vi "MeasurementLink Common Proto Generator.vi"(0 "Proto File Path":path[](array[path]), 1 "Generated Library Name":string, 2 "Library Suffix":string caption="Generated Library Suffix", 3 "Generate":enum16{"gRPC Server", "gRPC Client", "Both"}(ring), 5 "Import Paths":path[](array[path]), 7 "Prototype Library":path, 9 "Target Project":path, 11 "error in (no error)":errorcluster) -> (15 "error out":errorcluster)   [LabVIEW 2020]
uses:
  Generator/_Editor/MeasurementService Editor.lvlib
panel:
  in  "Debug - Prompt before deleting disk content? (F)":bool
  in  "Debug - Leave Project Open? (F)":bool
  # "Ignored for servers as of v0.5.2.2"
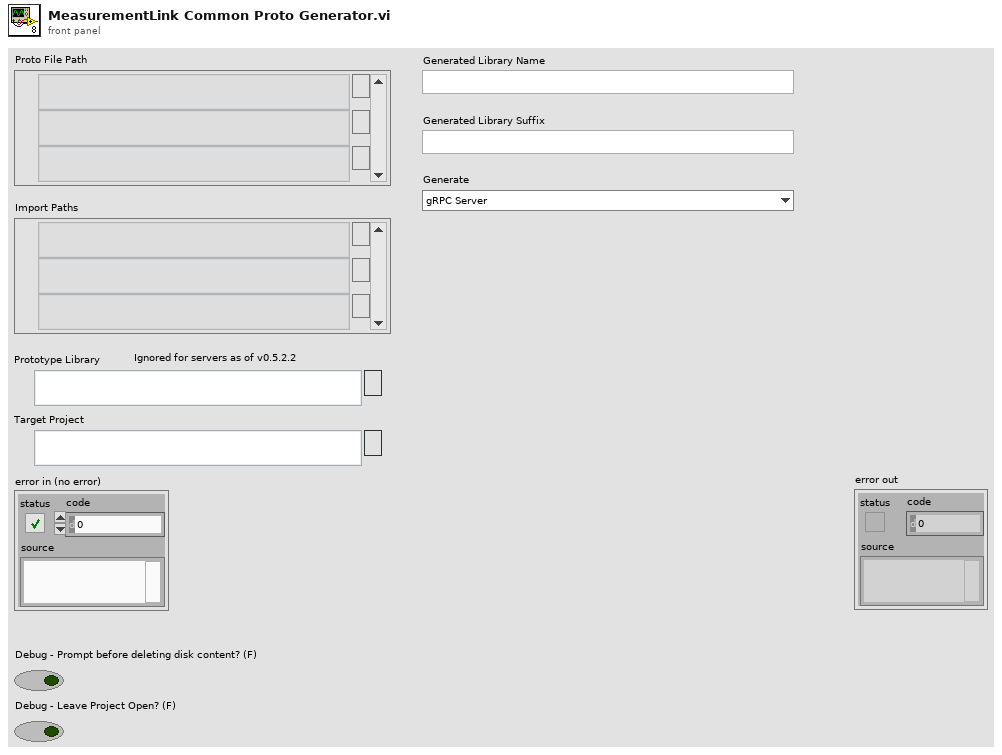
[diagram p1: front panel]
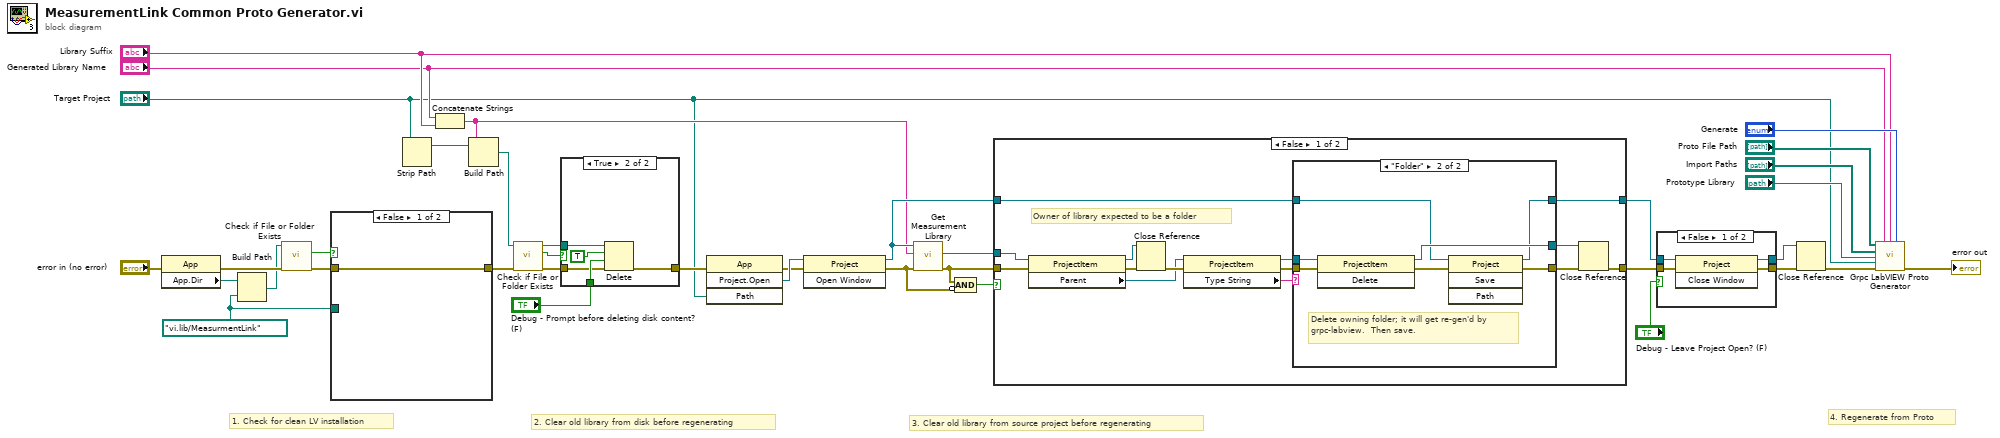
[diagram p0: block diagram]
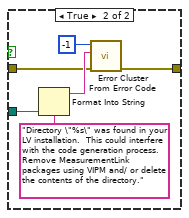
[diagram p2: hidden frame]
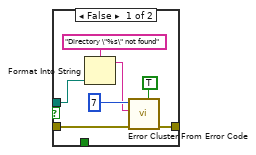
[diagram p3: hidden frame]
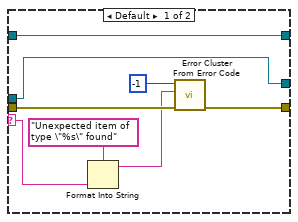
[diagram p4: hidden frame]
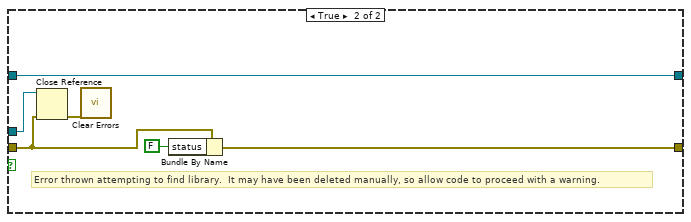
[diagram p5: hidden frame]
diagram:
  w1 = path "vi.lib/MeasurmentLink" ("Target Project")
  # "4. Regenerate from Proto"
  # "3. Clear old library from source project before regenerating"
  # "2. Clear old library from disk before regenerating"
  # "1. Check for clean LV installation"
  n1 = property class="App"(error in="error in (no error)") -> (error out=w6:errorcluster, "App.Dir"=w8:path)  [unwired: 1 in, 1 out]
  n2 = Build Path(base path=w8, name or relative path=w1) -> (appended path=w5:path)
  n3 = call <vilib>:"Check if File or Folder Exists.vi"("error in (no error)"=w6, "path"=w5) -> ("error out"=w3:errorcluster, "file or folder exists?"=w4:bool)  [unwired: 7 in, 1 out]
  n4 = case shown="False" w4 {
    tunnel: w3 -> [w38 w41]
    tunnel: [w38 w42] -> w2
    tunnel: w1 -> [_ w39]
    frame False {
    }
    frame True {
      n5 = Format Into String(format string="Directory \"%s\" was found in your LV installation.  This could interfere with the code generation process.  Remove MeasurementLink packages using VIPM and/ or delete the contents of the directory.", w39) -> (resulting string=w43:string)  [unwired: 2 in, 1 out]
      n6 = call <vilib>:"Error Cluster From Error Code.vi"("error in (no error)"=w41, "error message (\"\")"=w43, "error code (0)"=-1) -> ("error out"=w42:errorcluster)  [unwired: 6 in]
    }
  }
  n7 = Strip Path(path="Target Project") -> (stripped path=w10:path)  [unwired: 1 out]
  n8 = Concatenate Strings("Generated Library Name", "Library Suffix") -> (w26:string)
  n9 = Build Path(base path=w10, name or relative path=w26) -> (appended path=w22:path)
  n10 = call <vilib>:"Check if File or Folder Exists.vi"("error in (no error)"=w2, "path"=w22) -> ("error out"=w21:errorcluster, "file or folder exists?"=w19:bool, "dup path"=w20:path)  [unwired: 7 in]
  n11 = case shown="True" w19 {
    tunnel: [w50 w55] -> w25
    tunnel: "Debug - Prompt before deleting disk content? (F)" -> [_ w54]
    tunnel: w21 -> [w49 w53]
    tunnel: w20 -> [w47 w52]
    frame False {
      n12 = Format Into String(format string="Directory \"%s\" not found", w47) -> (resulting string=w46:string)  [unwired: 2 in, 1 out]
      n13 = call <vilib>:"Error Cluster From Error Code.vi"("is warning? (False)"=TRUE, "error in (no error)"=w49, "error message (\"\")"=w46, "error code (0)"=7) -> ("error out"=w50:errorcluster)  [unwired: 5 in]
    }
    frame True {
      n14 = Delete(path (use dialog)=w52, entire hierarchy (F)=TRUE, confirm (F)=w54, error in=w53) -> (error out=w55:errorcluster)  [unwired: 1 in, 2 out]
    }
  }
  n15 = invoke class="App" method="Project.Open"(error in=w25, "Path"="Target Project") -> (error out=w36:errorcluster, "Project:Open"=w37:refnum<vi>)  [unwired: 2 in, 2 out]
  n16 = invoke class="Project" method="Open Window"(reference=w37, error in=w36) -> (reference out=w27:refnum<vi>, error out=w29:errorcluster)  [unwired: 1 in, 1 out]
  n17 = call "Get Measurement Library.vi"("error in (no error)"=w29, "Measurement Service Name"=w26, "Project in"=w27) -> ("error out"=w23:errorcluster, "Measurement Library Item"=w28:refnum<vi>)  [unwired: 7 in]
  n18 = Compound Arithmetic op=AND(w23, invert w29) -> (w30:bool)
  n19 = case shown="False" w30 {
    tunnel: w28 -> [w69 w88]
    tunnel: w27 -> [w62 w89]
    tunnel: [w59 w89] -> w35
    tunnel: [w58 w91] -> w34
    tunnel: w23 -> [w57 w87]
    frame False {
      # "Owner of library expected to be a folder"
      n20 = property class="ProjectItem"(reference=w69, error in=w57) -> (reference out=w68:refnum<vi>, error out=w70:errorcluster, "Parent"=w66:refnum<vi>)
      n21 = Close Reference(reference=w68, error in (no error)=w70) -> (error out=w67:errorcluster)
      n22 = property class="ProjectItem"(reference=w66, error in=w67) -> (reference out=w63:refnum<vi>, error out=w64:errorcluster, "Type String"=w65:string)
      n23 = case shown="\"Folder\"" w65 {
        selector: w65 -> [w75 _]
        tunnel: w64 -> [w78 w85]
        tunnel: w63 -> [w72 w84]
        tunnel: [w77 w81] -> w61
        tunnel: w62 -> [w71 w80]
        tunnel: [w71 w79] -> w59
        tunnel: [w72 w83] -> w60
        frame Default {
          n24 = Format Into String(format string="Unexpected item of type \"%s\" found", w75) -> (resulting string=w74:string)  [unwired: 2 in, 1 out]
          n25 = call <vilib>:"Error Cluster From Error Code.vi"("error in (no error)"=w78, "error message (\"\")"=w74, "error code (0)"=-1) -> ("error out"=w77:errorcluster)  [unwired: 6 in]
        }
        frame "Folder" {
          # "Delete owning folder; it will get re-gen'd by grpc-labview.  Then save."
          n26 = invoke class="ProjectItem" method="Delete"(reference=w84, error in=w85) -> (reference out=w83:refnum<vi>, error out=w82:errorcluster)  [unwired: 1 in, 1 out]
          n27 = invoke class="Project" method="Save"(reference=w80, error in=w82) -> (reference out=w79:refnum<vi>, error out=w81:errorcluster)  [unwired: 2 in, 2 out]
        }
      }
      n28 = Close Reference(reference=w60, error in (no error)=w61) -> (error out=w58:errorcluster)
    }
    frame True {
      # "Error thrown attempting to find library.  It may have been deleted manually, so allow code to proceed with a warning."
      n29 = Close Reference(reference=w88, error in (no error)=w87) -> (error out=w86:errorcluster)
      n30 = call <vilib>:"Clear Errors.vi"("error in (no error)"=w86) -> ()  [unwired: 5 in, 2 out]
      n31 = Bundle By Name(cluster=w87, "status"=FALSE) -> (w91:errorcluster)
    }
  }
  n32 = case shown="False" "Debug - Leave Project Open? (F)" {
    tunnel: w35 -> [w95 w96]
    tunnel: w34 -> [w94 w97]
    tunnel: [w93 w97] -> w33
    tunnel: [w92 w96] -> w32
    frame False {
      n33 = invoke class="Project" method="Close Window"(reference=w95, error in=w94) -> (reference out=w92:refnum<vi>, error out=w93:errorcluster)  [unwired: 1 in, 1 out]
    }
    frame True {
    }
  }
  n34 = Close Reference(reference=w32, error in (no error)=w33) -> (error out=w18:errorcluster)
  n35 = call "Grpc LabVIEW Proto Generator.vi"("Proto File Path"="Proto File Path", "Generated Library Name"="Generated Library Name", "Library Suffix"="Library Suffix", "Generate"="Generate", "Import Paths"="Import Paths", "Prototype Library"="Prototype Library", "Target Project"="Target Project", "error in (no error)"=w18) -> ("error out"=→"error out":errorcluster)  [unwired: 7 in]
